vi "IdentificationGet.vi"(0 "SR865 in":T1, 5 "error in":errorcluster) -> (14 "SR865 out":T1, 16 "Identification":string, 19 "error out":errorcluster)   [LabVIEW 2018]
uses:
  SR865.ctl
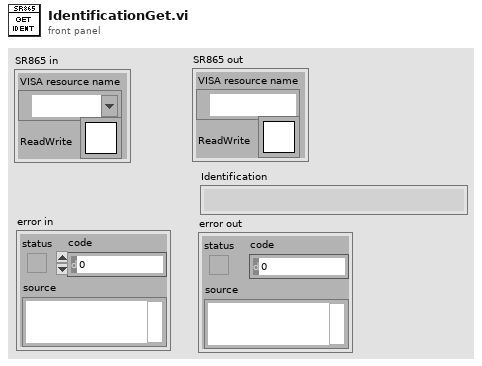
[diagram p1: front panel]
types:
  T1 = typedef "SR865.ctl" = cluster{"VISA resource name":refnum<visa-resource-name>, "ReadWrite":T2}
  T2 = typedef "Semaphore RefNum" = refnum<k1>
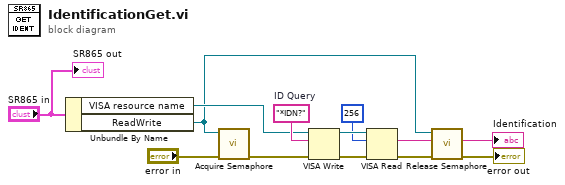
[diagram p0: block diagram]
diagram:
  w7 = "*IDN?"  # ID Query
  n1 = Unbundle By Name("SR865 in") -> ("VISA resource name"=w6:refnum<visa-resource-name>, "ReadWrite"=w1:T2)
  n2 = call <vilib>:"Acquire Semaphore.vi"("error in (no error)"="error in", "semaphore"=w1) -> ("error out"=w5:errorcluster)  [unwired: 3 in, 2 out]
  n3 = VISA Write(VISA resource name=w6, write buffer=w7, error in (no error)=w5) -> (VISA resource name out=w10:refnum<visa-resource-name>, error out=w9:errorcluster)  [unwired: 1 out]
  n4 = VISA Read(VISA resource name=w10, byte count=u32 256, error in (no error)=w9) -> (read buffer=→"Identification":string, error out=w3:errorcluster)  [unwired: 2 out]
  n5 = call <vilib>:"Release Semaphore.vi"("error in (no error)"=w3, "semaphore"=w1) -> ("error out"=→"error out":errorcluster)  [unwired: 4 in, 1 out]
  "SR865 out" <- "SR865 in"
